vi "Bai1_5.vi"() -> ()   [LabVIEW 2023]
panel:
  out "Array 2":dbl[](array[numeric])
  in  "Cluster 2":T1
  in  "stop":bool
  out "Cluster":T1
  in  "Array":dbl[](array[numeric])
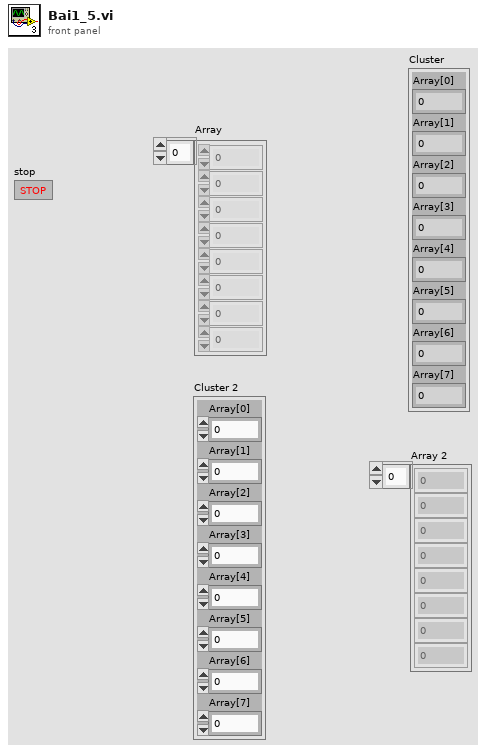
[diagram p1: front panel]
types:
  T1 = cluster{"Array[0]":dbl, "Array[1]":dbl, "Array[2]":dbl, "Array[3]":dbl, "Array[4]":dbl, "Array[5]":dbl, "Array[6]":dbl, "Array[7]":dbl}
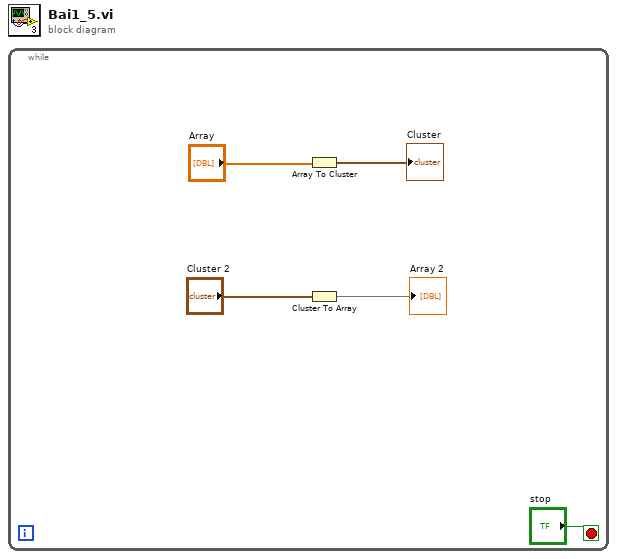
[diagram p0: block diagram]
diagram:
  n1 = while {
    stop <- "stop" stop-if-true
    n2 = Array To Cluster(array="Array") -> (cluster=→"Cluster":T1)
    n3 = Cluster To Array(cluster="Cluster 2") -> (array=→"Array 2":dbl[])
  }
